vi "Simulated Console.vi"(8 "error in (no error)":errorcluster) -> (0 "error out":errorcluster)   [LabVIEW 2011]
doc: "[Covers: UI1]"
uses:
  Keypad/Keypad.xctl
  TypeDefs/CTRL to UI Message.ctl
  TypeDefs/CTRL to UI Command.ctl
  TypeDefs/UI to CTRL Message.ctl
  TypeDefs/UI to CTRL Command.ctl
  TypeDefs/User Console Commands.ctl
  TypeDefs/Error Classification.ctl
  TypeDefs/UI Items.ctl
panel:
  in  "Keypad":i32(xcontrol)
  in  "Right Button 3":bool
  in  "Right Button 2":bool
  in  "Right Button 1":bool
  out "Right Menu 3":string
  out "Right Menu 2":string
  out "Right Menu 1":string
  out "Left Menu 3":string
  out "Left Menu 2":string
  out "Left Menu 1":string
  in  "Left Button 3":bool
  in  "Left Button 2":bool
  in  "Left Button 1":bool
  out "ATM Messages":string
  in  "Card Slot":bool
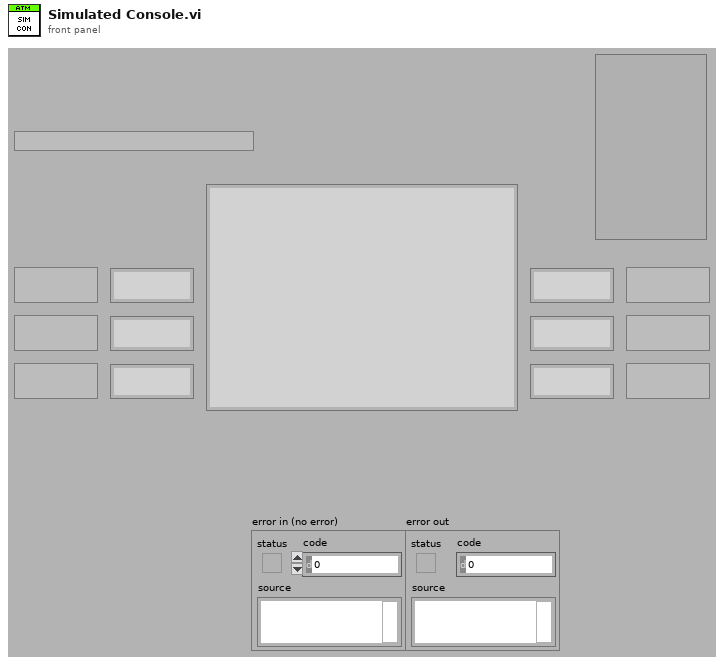
[diagram p1: front panel]
types:
  T1 = typedef "User Console Commands.ctl" = enum16{"Init", "Set ATM Message", "Set ATM Menus", "Disable Controls", "Wait for Input", "Clear Keypad", "Return Card", "Close"}
  T2 = typedef "UI to CTRL Message.ctl" = cluster{"Command":T3, "Data":variant}
  T3 = typedef "UI to CTRL Command.ctl" = enum16{"Card Inserted", "Keypad Entry", "Button Pressed"}
  T4 = typedef "CTRL to UI Message.ctl" = cluster{"Command":T5, "Data":variant}
  T5 = typedef "CTRL to UI Command.ctl" = enum16{"Display Message", "Return Card", "Stop", "Set Menu", "Clear Keypad", "Disable UI Elements"}
  T6 = typedef "Error Classification.ctl" = enum16{"Minor", "Session", "System"}
  T7 = typedef "UI Items.ctl" = cluster{"Keypad":bool, "Card Slot":bool, "Left Buttons":bool, "Right Buttons":bool, "ATM Message":bool, "Left Menu":bool, "Right Menu":bool}
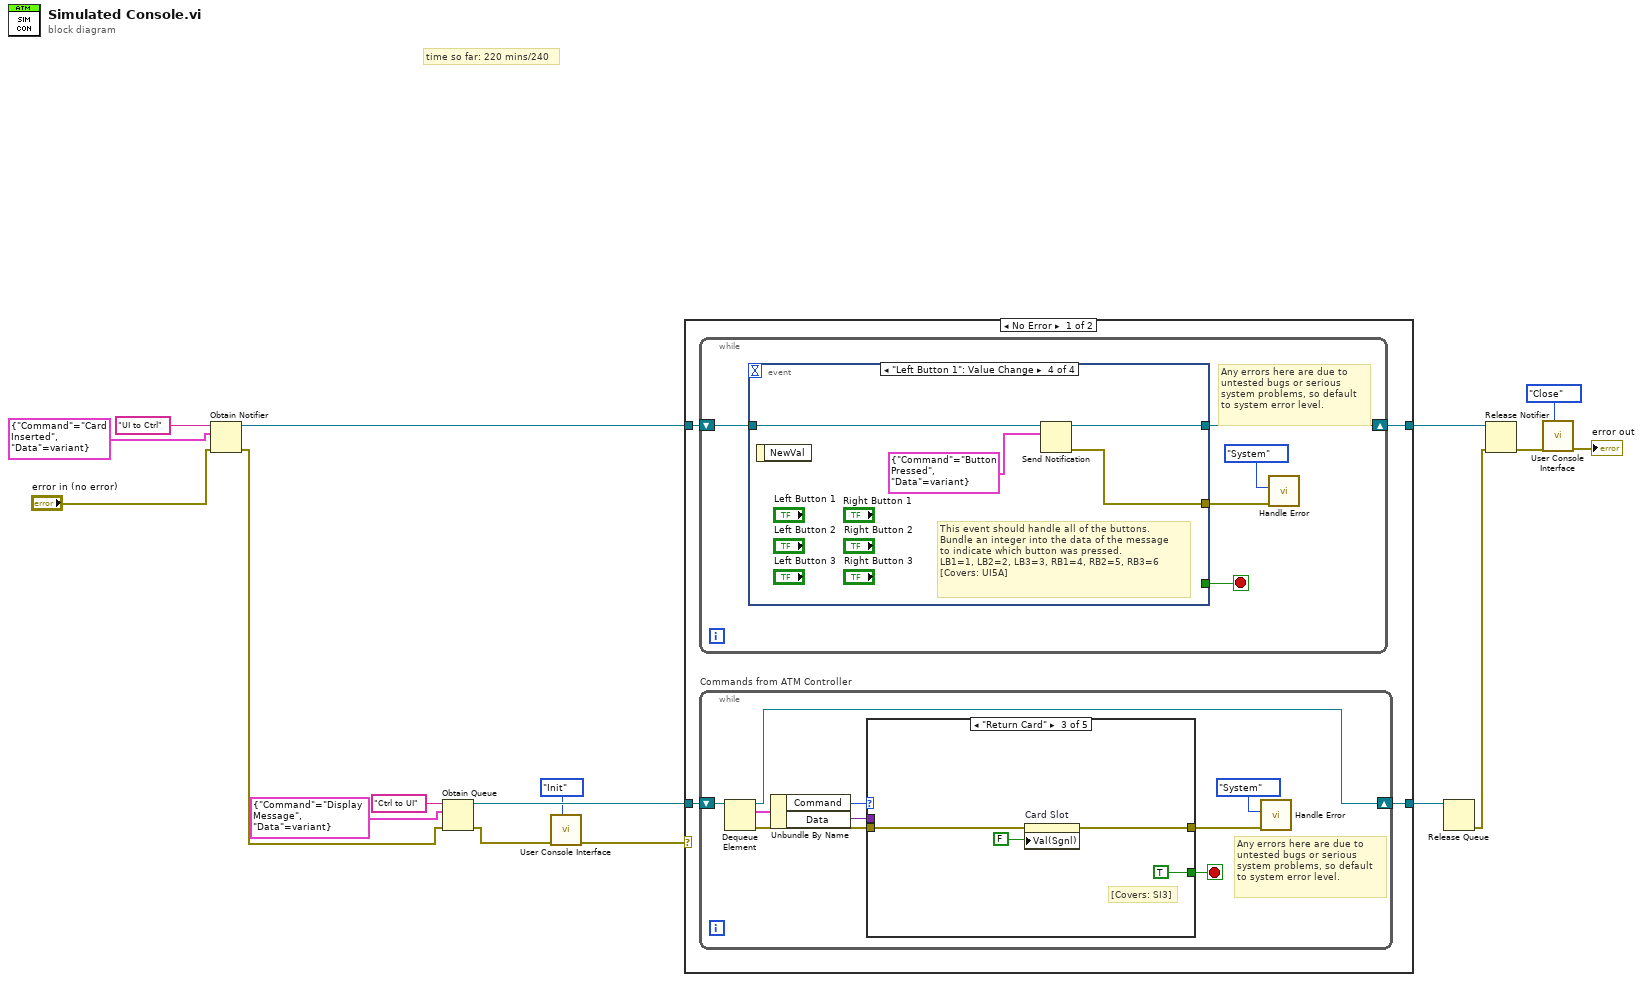
[diagram p0: block diagram]
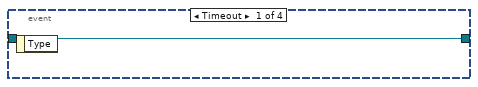
[diagram p2: hidden frame]
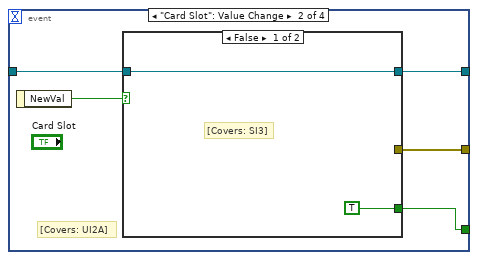
[diagram p3: hidden frame]
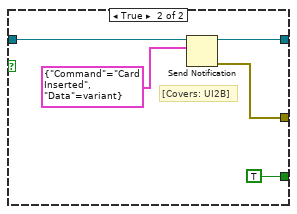
[diagram p4: hidden frame]
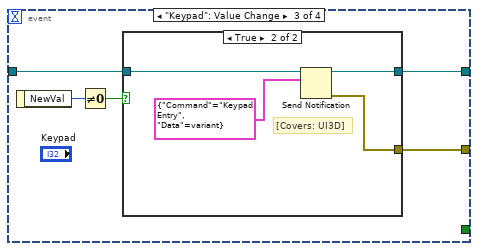
[diagram p5: hidden frame]
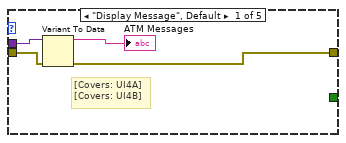
[diagram p7: hidden frame]
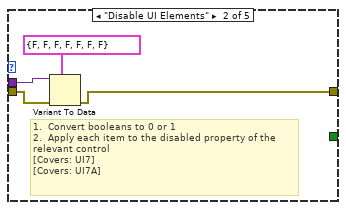
[diagram p8: hidden frame]
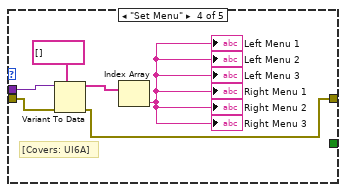
[diagram p9: hidden frame]
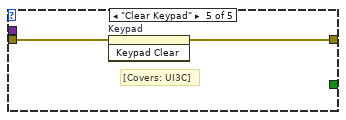
[diagram p10: hidden frame]
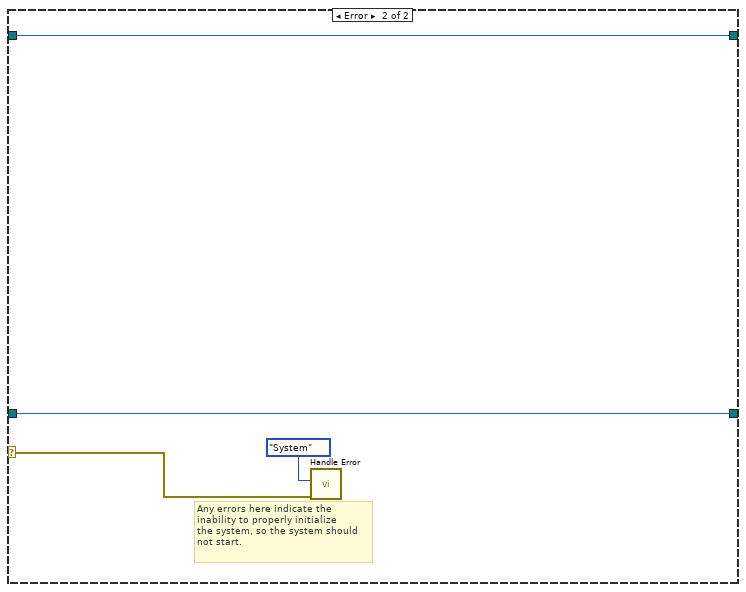
[diagram p11: hidden frame]
diagram:
  # "time so far: 220 mins/240"
  n1 = Obtain Notifier(name (unnamed)="UI to Ctrl", notification data type=T2 {"Command"=enum."Card Inserted", "Data"=variant} ("Cluster"), error in (no error)="error in (no error)") -> (notifier out=w12:refnum<notifier>, error out=w7:errorcluster)  [unwired: 1 in, 1 out]
  n2 = Obtain Queue(name (unnamed)="Ctrl to UI", element data type=T4 {"Command"=enum."Display Message", "Data"=variant} ("Cluster"), error in (no error)=w7) -> (queue out=w15:refnum<queue>, error out=w6:errorcluster)  [unwired: 2 in, 1 out]
  n3 = call "User Console Interface.vi"("Command"=User_Console_Commands."Init", "error in (no error)"=w6) -> ("error out"=w5:errorcluster)  [unwired: 6 in, 3 out]
  n4 = case shown="No Error" w5 {
    selector: w5 -> [_ w85]
    tunnel: w15 -> [w21 w83]
    tunnel: w12 -> [w20 w84]
    tunnel: [w19 w84] -> w9
    tunnel: [w18 w83] -> w10
    frame No Error {
      n5 = while {
        shift-right: [w22] -> w19
        shift-left: w20 -> [w25]
        stop <- w26 stop-if-true
        # "Any errors here are due to\nuntested bugs or serious\nsystem problems, so default\nto system error level."
        n6 = event shown="[3] \"Left Button 1\": Value Change" {
          selector: _ -> [_ _ _ _]
          dyn-events: _ -> [_ _ _ _]
          timeout: _ -> [_ _ _ _]
          tunnel: [_ w28 _ _] -> w26
          tunnel: w25 -> [w27 w32 w44 w53]
          tunnel: [_ w30 w43 w52] -> w23
          tunnel: [w27 w29 w42 w51] -> w22
          event Timeout {
            n7 = event-data() -> ()  [unwired: 1 in, 1 out]
          }
          event "Card Slot": Value Change {
            # "[Covers: UI2A]"
            n8 = event-data() -> ("NewVal"=w31:bool)  [unwired: 1 in]
            n9 = case shown="False" w31 {
              tunnel: w32 -> [w34 w39]
              tunnel: [_ w37] -> w30
              tunnel: [w34 w36] -> w29
              tunnel: [TRUE ("Stop") TRUE ("Stop")] -> w28
              frame False {
                # "[Covers: SI3]"
              }
              frame True {
                # "[Covers: UI2B]"
                n10 = Send Notification(notification=T2 {"Command"=enum."Card Inserted", "Data"=variant}, notifier=w39) -> (notifier out=w36:refnum<notifier>, error out=w37:errorcluster)  [unwired: 1 in]
              }
            }
          }
          event "Keypad": Value Change {
            n11 = event-data() -> ("NewVal"=w41:i32)  [unwired: 1 in]
            n12 = Not Equal To 0?(x=w41) -> (x != 0?=w40:bool)
            n13 = case shown="True" w40 {
              tunnel: w44 -> [w45 w49]
              tunnel: [_ w47] -> w43
              tunnel: [w45 w46] -> w42
              frame False {
                # "Ignoring zero values prevents messages when\nclearing the keypad and also prevents the user\nfrom entering 0 for a deposit or withdrawal as\nthe reaction to that situation isn't defined by\nthe requirements."
              }
              frame True {
                # "[Covers: UI3D]"
                n14 = Send Notification(notification=T2 {"Command"=enum."Keypad Entry", "Data"=variant}, notifier=w49) -> (notifier out=w46:refnum<notifier>, error out=w47:errorcluster)  [unwired: 1 in]
              }
            }
          }
          event "Left Button 1": Value Change {
            # "This event should handle all of the buttons.\nBundle an integer into the data of the message \nto indicate which button was pressed.\nLB1=1, LB2=2, LB3=3, RB1=4, RB2=5, RB3=6\n[Covers: UI5A]"
            n15 = event-data() -> ()  [unwired: 1 in, 1 out]
            n16 = Send Notification(notification=T2 {"Command"=enum."Button Pressed", "Data"=variant}, notifier=w53) -> (notifier out=w51:refnum<notifier>, error out=w52:errorcluster)  [unwired: 1 in]
          }
        }
        n17 = call "Handle Error.vi"("error in (no error)"=w23, "Classification"=Error_Classification."System") -> ()  [unwired: 7 in, 3 out]
      }
      n18 = while "Commands from ATM Controller" {
        shift-right: [w54] -> w18
        shift-left: w21 -> [w62]
        stop <- w58 stop-if-true
        # "Any errors here are due to\nuntested bugs or serious\nsystem problems, so default\nto system error level."
        n19 = Dequeue Element(queue=w62) -> (queue out=w54:refnum<queue>, element=w61:T4, error out=w57:errorcluster)  [unwired: 2 in, 1 out]
        n20 = Unbundle By Name(w61) -> ("Command"=w60:T5, "Data"=w59:variant)
        n21 = case shown="\"Return Card\"" w60 {
          tunnel: w59 -> [w66 w70 _ w80 _]
          tunnel: [_ _ TRUE _ _] -> w58
          tunnel: w57 -> [w65 w69 w73 w78 w82]
          tunnel: [w63 w67 w72 w75 w81] -> w56
          frame "Display Message", Default {
            # "[Covers: UI4A]\n[Covers: UI4B]"
            n22 = Variant To Data(error in=w65, Variant=w66) -> (data=→"ATM Messages":string, error out=w63:errorcluster)  [unwired: 1 in]
          }
          frame "Disable UI Elements" {
            # "1.  Convert booleans to 0 or 1\n2.  Apply each item to the disabled property of the\nrelevant control\n[Covers: UI7]\n[Covers: UI7A]"
            n23 = Variant To Data(error in=w69, type=T7 {"Keypad"=FALSE, "Card Slot"=FALSE, "Left Buttons"=FALSE, "Right Buttons"=FALSE, "ATM Message"=FALSE, "Left Menu"=FALSE, "Right Menu"=FALSE} ("UI Items"), Variant=w70) -> (error out=w67:errorcluster)  [unwired: 1 out]
          }
          frame "Return Card" {
            # "[Covers: SI3]"
            n24 = property on="Card Slot" class="Bool (strict)"(error in=w73, "Val(Sgnl)"=FALSE ("Value (Signaling)")) -> (error out=w72:errorcluster)  [unwired: 1 in, 1 out]
          }
          frame "Set Menu" {
            # "[Covers: UI6A]"
            n25 = Variant To Data(error in=w78, type=string[] [], Variant=w80) -> (data=w77:string[], error out=w75:errorcluster)
            n26 = Index Array(array=w77) -> (element=→"Left Menu 1" →"Left Menu 2" →"Left Menu 3" →"Right Menu 1" →"Right Menu 2" →"Right Menu 3":string)  [unwired: 1 in]
          }
          frame "Clear Keypad" {
            # "[Covers: UI3C]"
            n27 = invoke on="Keypad" class="Keypad (strict)" method="Keypad Clear"(error in=w82) -> (error out=w81:errorcluster)  [unwired: 2 in, 2 out]
          }
        }
        n28 = call "Handle Error.vi"("error in (no error)"=w56, "Classification"=Error_Classification."System") -> ()  [unwired: 7 in, 3 out]
      }
    }
    frame Error {
      # "Any errors here indicate the\ninability to properly initialize\nthe system, so the system should\nnot start."
      n29 = call "Handle Error.vi"("error in (no error)"=w85, "Classification"=Error_Classification."System") -> ()  [unwired: 7 in, 3 out]
    }
  }
  n30 = Release Queue(queue=w10) -> (error out=w8:errorcluster)  [unwired: 2 in, 2 out]
  n31 = Release Notifier(notifier=w9, error in (no error)=w8) -> (error out=w2:errorcluster)  [unwired: 1 in, 2 out]
  n32 = call "User Console Interface.vi"("Command"=User_Console_Commands."Close", "error in (no error)"=w2) -> ("error out"=→"error out":errorcluster)  [unwired: 6 in, 3 out]
